vi "Dopocet_presne_nuly.vi"(8 "dt":dbl, 11 "Vstupní pole":dbl[](array[numeric])) -> (2 "XY Graph":cluster{dbl[], "Vstupní pole":dbl[]}(graph))   [LabVIEW 2019]
panel:
  out "y array 2":dbl[](array[numeric])
  out "x array":dbl[](array[numeric])
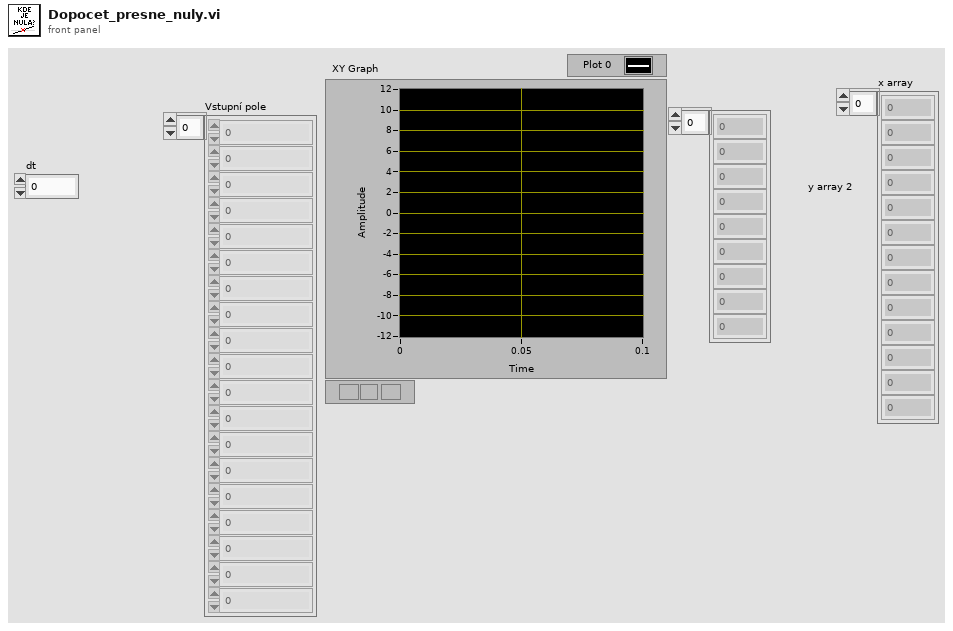
[diagram p1: front panel]
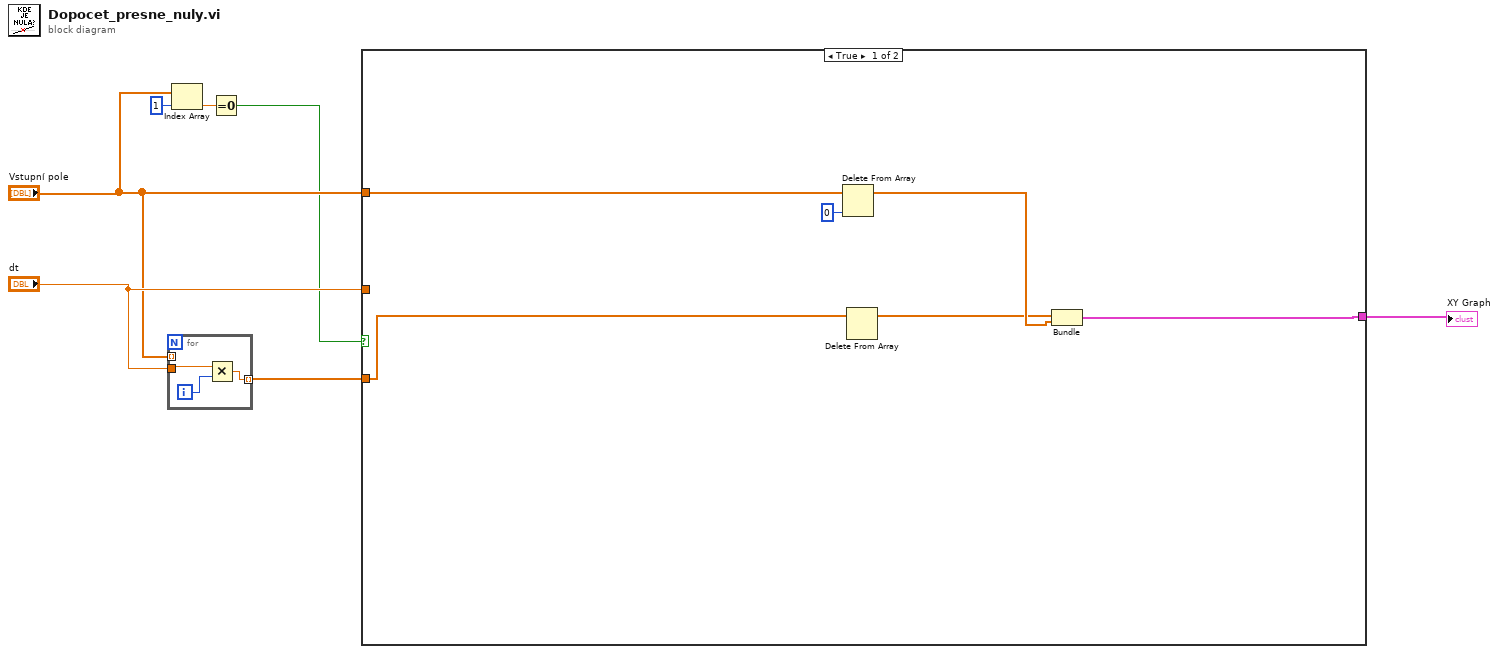
[diagram p0: block diagram]
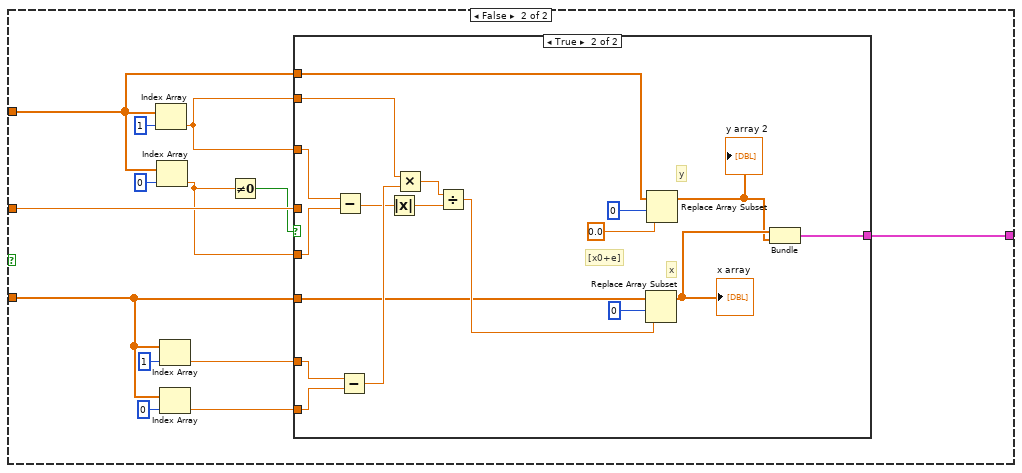
[diagram p2: hidden frame]
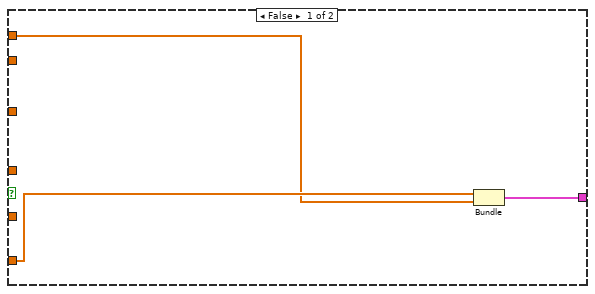
[diagram p3: hidden frame]
diagram:
  n1 = for {
    tunnel: "dt" -> [w9]
    tunnel: "Vstupní pole" -> [_] mode=indexing
    tunnel: [w8] -> w6 mode=indexing
    i -> [w10]
    n2 = Multiply(x=w9, y=w10) -> (x*y=w8:dbl)
  }
  n3 = Index Array(array="Vstupní pole", index=1) -> (element=w3:dbl)
  n4 = Equal To 0?(x=w3) -> (x = 0?=w2:bool)
  n5 = case shown="True" w2 {
    tunnel: "dt" -> [_ w27]
    tunnel: w6 -> [w13 w22]
    tunnel: "Vstupní pole" -> [w16 w18]
    tunnel: [w11 w17] -> w1
    frame True {
      n6 = Delete From Array(array=w16, index=0) -> (array with subset deleted=w15:dbl[])  [unwired: 1 in, 1 out]
      n7 = Delete From Array(array=w13) -> (array with subset deleted=w12:dbl[])  [unwired: 2 in, 1 out]
      n8 = Bundle(w12, "Vstupní pole"=w15) -> (w11:cluster{dbl[], "Vstupní pole":dbl[]})  [unwired: 1 in]
    }
    frame False {
      n9 = Index Array(array=w18, index=1) -> (element=w19:dbl)
      n10 = Index Array(array=w18, index=0) -> (element=w26:dbl)
      n11 = Index Array(array=w22, index=1) -> (element=w21:dbl)
      n12 = Index Array(array=w22, index=0) -> (element=w20:dbl)
      n13 = Not Equal To 0?(x=w26) -> (x != 0?=w25:bool)
      n14 = case shown="True" w25 {
        tunnel: w19 -> [_ w44]
        tunnel: w26 -> [_ w43]
        tunnel: w27 -> [_ _]
        tunnel: w19 -> [_ w35]
        tunnel: w22 -> [w32 w36]
        tunnel: w21 -> [_ w45]
        tunnel: w20 -> [_ w42]
        tunnel: [w31 w38] -> w17
        tunnel: w18 -> [w30 w37]
        frame False {
          n15 = Bundle(w32, "Vstupní pole"=w30) -> (w31:cluster{dbl[], "Vstupní pole":dbl[]})  [unwired: 1 in]
        }
        frame True {
          # "x"
          # "y"
          # "[x0+e]"
          n16 = Subtract(x=w44, y=w43) -> (x-y=w33:dbl)
          n17 = Subtract(x=w45, y=w42) -> (x-y=w41:dbl)
          n18 = Absolute Value(x=w33) -> (abs(x)=w34:dbl)
          n19 = Multiply(x=w35, y=w41) -> (x*y=w40:dbl)
          n20 = Divide(x=w40, y=w34) -> (x/y=w39:dbl)
          n21 = Replace Array Subset(array=w36, new element=w39, index=0) -> (w47:dbl[])
          "x array" <- w47
          n22 = Replace Array Subset(array=w37, new element=0.0, index=0) -> (w46:dbl[])
          "y array 2" <- w46
          n23 = Bundle(w47, "Vstupní pole"=w46) -> (w38:cluster{dbl[], "Vstupní pole":dbl[]})  [unwired: 1 in]
        }
      }
    }
  }
  "XY Graph" <- w1
